vi "Pre Launch Init.vi"(11 "EventLog in":refnum<class "EventLog.lvclass">) -> (0 "error out":errorcluster, 3 "EventLog out":refnum<class "EventLog.lvclass">)   [LabVIEW 2019, in "EventLog.lvlib" / "EventLog.lvclass"]
doc: "(<B>Filename</B>: Actor Framework.lvlib:Actor.lvclass:Pre Launch Init.vi)\n\nDefines behavior that occurs after the Launch Nested Actor method is invoked but before the actor's Actor Core method begins running.\n\nBy default, this method does nothing. A descendant class may override it to define behavior."
uses:
  EventLog.lvclass
  C:/Projekty/_Wewnetrzne/PC_ActorFramework/07_Program/LABVIEW/02_Source/SubModules/LogsAbstract/LogsAbstract.lvclass
  C:/Program Files (x86)/National Instruments/LabVIEW 2019/vi.lib/ActorFramework/Actor/Actor.lvclass
  TypeDef/EventLog Header.ctl
  LogsAbstract/TypeDef/Event Source.ctl
  <vilib>/ActorFramework/Actor/Actor.lvclass/Actor.ctl
  <vilib>/ActorFramework/Message Enqueuer/Message Enqueuer.lvclass/Message Enqueuer.ctl
  EventLog.lvclass/EventLog.ctl
  <vilib>/ActorFramework/Message Enqueuer/Init from Existing Queue.vi
  FGV+Globals/EventLogRef Global.vi
  Classes/Event/sVI/Predefinied Events/StartApp Event.vi
  LogsAbstract/LogsAbstract.lvclass
  <vilib>/ActorFramework/Message Enqueuer/Message Enqueuer.lvclass
  Classes/Event/Event.lvclass
  <vilib>/ActorFramework/Actor/Actor.lvclass
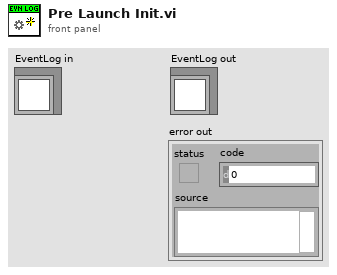
[diagram p1: front panel]
types:
  T1 = typedef "LogsAbstract.lvlib/LogsAbstract.lvclass/Event Source.ctl" = enum16{"LabView Call Chain", "Unknown", "< --- Modules --- >", "Core", "< --- SubModules --- >", "EventLog -> Core", "ErrorLog -> Core"}
  T2 = typedef "EventLog.lvlib/EventLog.lvclass/EventLog Header.ctl" = string[]
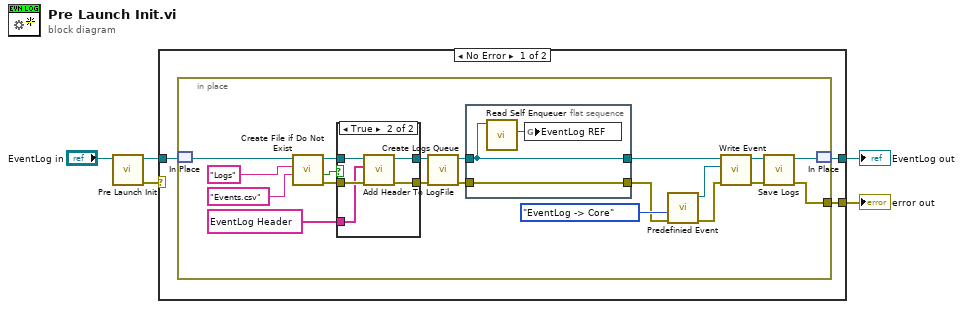
[diagram p0: block diagram]
diagram:
  n1 = call-parent "Pre Launch Init.vi"("LogsAbstract in"="EventLog in") -> ("error out"=w1:errorcluster, "LogsAbstract out"=w2:refnum<class "EventLog.lvclass">)  [unwired: 9 in]
  n2 = case shown="No Error" w1 {
    selector: w1 -> [_ w40]
    tunnel: [w8 w39] -> w5
    tunnel: [w7 w40] -> w4
    tunnel: w2 -> [w6 w39]
    frame No Error {
      n3 = in-place {
        in-place-border: [w18] -> w7
        n4 = in-place-match #1(w6) -> (w16:refnum<class "EventLog.lvclass">)
        n5 = call "Create File if Do Not Exist.vi"("FileName"="Events.csv", "FolderName"="Logs", "LogsClass In"=w16) -> ("ErrorOut"=w26:errorcluster, "File Created?"=w27:bool, "LogClass Out"=w28:refnum<class "EventLog.lvclass">)  [unwired: 6 in]
        n6 = case shown="True" w27 {
          tunnel: w28 -> [w32 w38]
          tunnel: w26 -> [w33 w37]
          tunnel: [w32 w36] -> w22
          tunnel: [w33 w35] -> w21
          tunnel: T2 ["Date", "Time", "Description", "Classification", "Origin", "Comment"] ("Eventlog Header") -> [_ w34]
          frame False {
          }
          frame True {
            n7 = call "Add Header To LogFile.vi"("Error In"=w37, "Header"=w34, "LogClass In"=w38) -> ("Error Out"=w35:errorcluster, "LogClass Out"=w36:refnum<class "EventLog.lvclass">)  [unwired: 7 in]
          }
        }
        n8 = call-dynamic "Create Logs Queue.vi"("Error In"=w21, "EventLog in"=w22) -> ("Error Out"=w14:errorcluster, "EventLog out"=w15:refnum<class "EventLog.lvclass">)  [unwired: 8 in]
        n9 = flat-sequence {
          tunnel: w15 -> [w29]
          tunnel: w14 -> [w30]
          tunnel: [w30] -> w13
          tunnel: [w29] -> w11
          frame #0 {
            n10 = call <vilib>:"Read Self Enqueuer.vi"("Actor"=w29) -> ("Self Enqueuer"=w31:refnum<class "Message Enqueuer.lvclass">)  [unwired: 10 in]
            n11 = global write "EventLogRef Global.vi" "EventLog REF"(w31) -> ()
          }
        }
        n12 = call-poly "Predefinied Event.vi"("error in (no error)"=w13, "Source"=Event_Source."EventLog -> Core" ("Origin")) -> ("error out"=w20:errorcluster, "Events out"=w9:refnum<class "Event.lvclass">)  [unwired: 8 in]
        n13 = call "Write Event.vi"("error in (no error)"=w20, "Event.lvclass"=w9, "EventLog in"=w11) -> ("error out"=w12:errorcluster, "EventLog out"=w10:refnum<class "EventLog.lvclass">)  [unwired: 7 in]
        n14 = call-dynamic "Save Logs.vi"("Error In"=w12, "EventLog in"=w10) -> ("Error Out"=w18:errorcluster, "EventLog out"=w19:refnum<class "EventLog.lvclass">)  [unwired: 8 in]
        n15 = in-place-match #1(w19) -> (w8:refnum<class "EventLog.lvclass">)
      }
    }
    frame Error {
    }
  }
  "error out" <- w4
  "EventLog out" <- w5
